vi "Teleop.vi"(10 "Match Info":T1={"Autonomous Elapsed Seconds"=0.0, "TeleOp Elapsed Seconds"=0.0, "Disabled Elapsed Seconds"=0.0, "Visited Autonomous"=FALSE, "Visited TeleOp"=FALSE, "Visited Disabled"=FALSE, "Autonomous Settings"={"Autonomous Style"=enum."Independent", "VI Refnum"=refnum}}, 11 "Call Context":T2) -> ()   [LabVIEW 2013]
doc: "This VI is called for each TeleOp packet received from the DS where the robot is not disabled. It is often used to read from the joysticks and update I/O or to update setpoints for timed control loops. It should complete and return within 20 milliseconds or it may miss DS packets."
uses:
  <vilib>/Rock Robotics/WPI/DriverStation/WPI_DriverStationDerivedRobotMode.ctl
  <vilib>/Rock Robotics/WPI/DriverStation/WPI_DriverStationMatch Info.ctl
  Robot Global Data.vi
  <vilib>/Rock Robotics/WPI/Solenoid/Deprecated/WPI_SolenoidSetBool.vi
  Angle.vi
  <vilib>/Rock Robotics/WPI/Joystick/WPI_JoystickGetSetRefNum.vi
  <vilib>/Rock Robotics/WPI/RobotDrive/WPI_RobotDriveGetSetRefNum.vi
panel:
  in  "Speed":dbl=0.5 format="%#_13g"
  out "Distance 2":dbl
  out "Rate 2":dbl
  out "Rate 1":dbl
  out "Distance 1":dbl
  out "Numeric 1":dbl(slide) scale=0.0..100.0
  out "Boolean 2":bool
  out "Boolean 1":bool
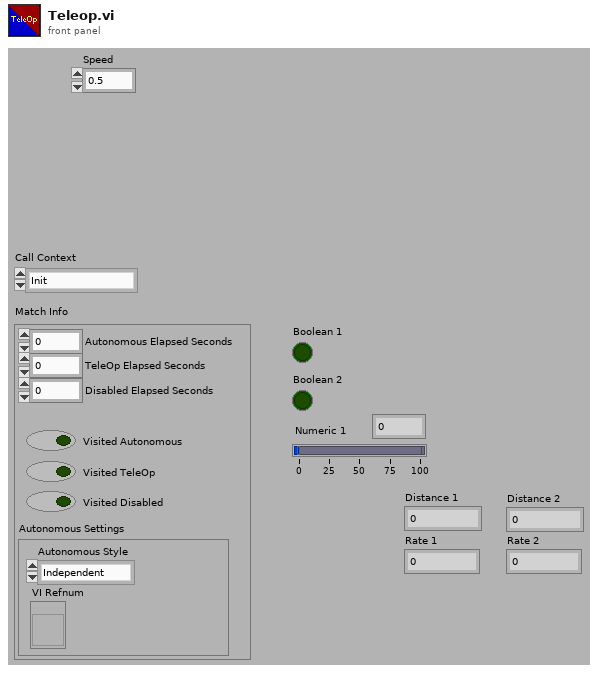
[diagram p1: front panel]
types:
  T1 = typedef "WPI_DriverStationMatch Info.ctl" = cluster{"Autonomous Elapsed Seconds":dbl, "TeleOp Elapsed Seconds":dbl, "Disabled Elapsed Seconds":dbl, "Visited Autonomous":bool, "Visited TeleOp":bool, "Visited Disabled":bool, "Autonomous Settings":cluster{"Autonomous Style":enum16{"Iterative", "Independent"}, "VI Refnum":refnum<vi>}}
  T2 = typedef "WPI_DriverStationDerivedRobotMode.ctl" = enum16{"Init", "Execute", "Stop"}
  T3 = typedef "WPI_RobotDriveDevRef.ctl" = cluster{"DevStatus":errorcluster, "Motors[]":T4[], "Square Inputs":bool, "Max Output":dbl, "Isochronous":bool}
  T4 = typedef "WPI_MotorControlDeviceRef.ctl" = cluster{"DeviceStatus":errorcluster, "Type":enum16{"PWM", "CAN"}, "PWM":cluster{"Digital Module":T5, "PWM Channel":T6, "DeadBand":T7}, "CAN":cluster{"Device Number":u8, "Control Mode":T8, "Semaphore":T9, "Max Vout":dbl}, "Invert":bool, "TransformRef":T10, "InvTransformRef":T10}
  T5 = typedef "FPGA_TypedefDigitalModule.ctl" = enum16{"Digital Module 1", "Digital Module 2"}
  T6 = typedef "FPGA_DIOPWMChannel.ctl" = enum8{"PWM 1", "PWM 2", "PWM 3", "PWM 4", "PWM 5", "PWM 6", "PWM 7", "PWM 8", "PWM 9", "PWM 10", "Invalid"}
  T7 = typedef "WPI_PWMDeadband.ctl" = cluster{"Name":string, "maxPositivePwm":i32, "minPositivePwm":i32, "centerPwm":i32, "maxNegativePwm":i32, "minNegativePwm":i32, "angularRange":u16}
  T8 = typedef "WPI_CANJaguar_ControlMode.ctl" = enum8{"Percent VBus", "Current", "Speed", "Position", "Voltage"}
  T9 = typedef "Semaphore RefNum" = refnum<k1>
  T10 = typedef "WPI_PWMTransform_ConPane.ctl" = refnum<vi>
  T11 = typedef "WPI_JoystickDevRef.ctl" = cluster{"Device":T12}
  T12 = typedef "WPI_JoystickDeviceEnum.ctl" = enum16{"USB 1", "USB 2", "USB 3", "USB 4", "Kinect 1", "Kinect 2"}
  T13 = typedef "WPI_JoystickButtonState.ctl" = cluster{"Button 1":bool, "Button 2":bool, "Button 3":bool, "Button 4":bool, "Button 5":bool, "Button 6":bool, "Button 7":bool, "Button 8":bool, "Button 9":bool, "Button 10":bool, "Button 11":bool, "Button 12":bool}
  T14 = cluster{"axis 1 (x)":dbl, "axis 2 (y)":dbl, "axis 3 (throttle)":dbl, "axis 4":dbl, "axis 5":dbl, "axis 6":dbl}
  T15 = typedef "WPI_SolenoidDevRef.ctl" = cluster{"DevStatus":errorcluster, "Solenoid Module":T16, "Forward Solenoid Channel":T17, "Reverse Solenoid Channel":T17}
  T16 = typedef "FPGA_TypedefSolenoidModule.ctl" = enum16{"Solenoid Module 1", "Solenoid Module 2"}
  T17 = typedef "WPI_SolenoidChannel.ctl" = enum8{"Solenoid 1", "Solenoid 2", "Solenoid 3", "Solenoid 4", "Solenoid 5", "Solenoid 6", "Solenoid 7", "Solenoid 8", "Invalid"}
  T18 = typedef "WPI_EncoderDevRef.ctl" = cluster{"DevStatus":errorcluster, "EncoderIndex":T19, "CounterIndex":T20, "DistancePerCount":dbl, "Decoding Type":T21}
  T19 = typedef "FPGA_EncoderIdx.ctl" = enum8{"Enc 0", "Enc 1", "Enc 2", "Enc 3", "Invalid"}
  T20 = typedef "FPGA_CounterCtrSystemIndex.ctl" = enum8{"Ctr 0", "Ctr 1", "Ctr 2", "Ctr 3", "Ctr 4", "Ctr 5", "Ctr 6", "Ctr 7", "Invalid"}
  T21 = typedef "WPI_EncoderType.ctl" = enum16{"1x", "2x", "4x"}
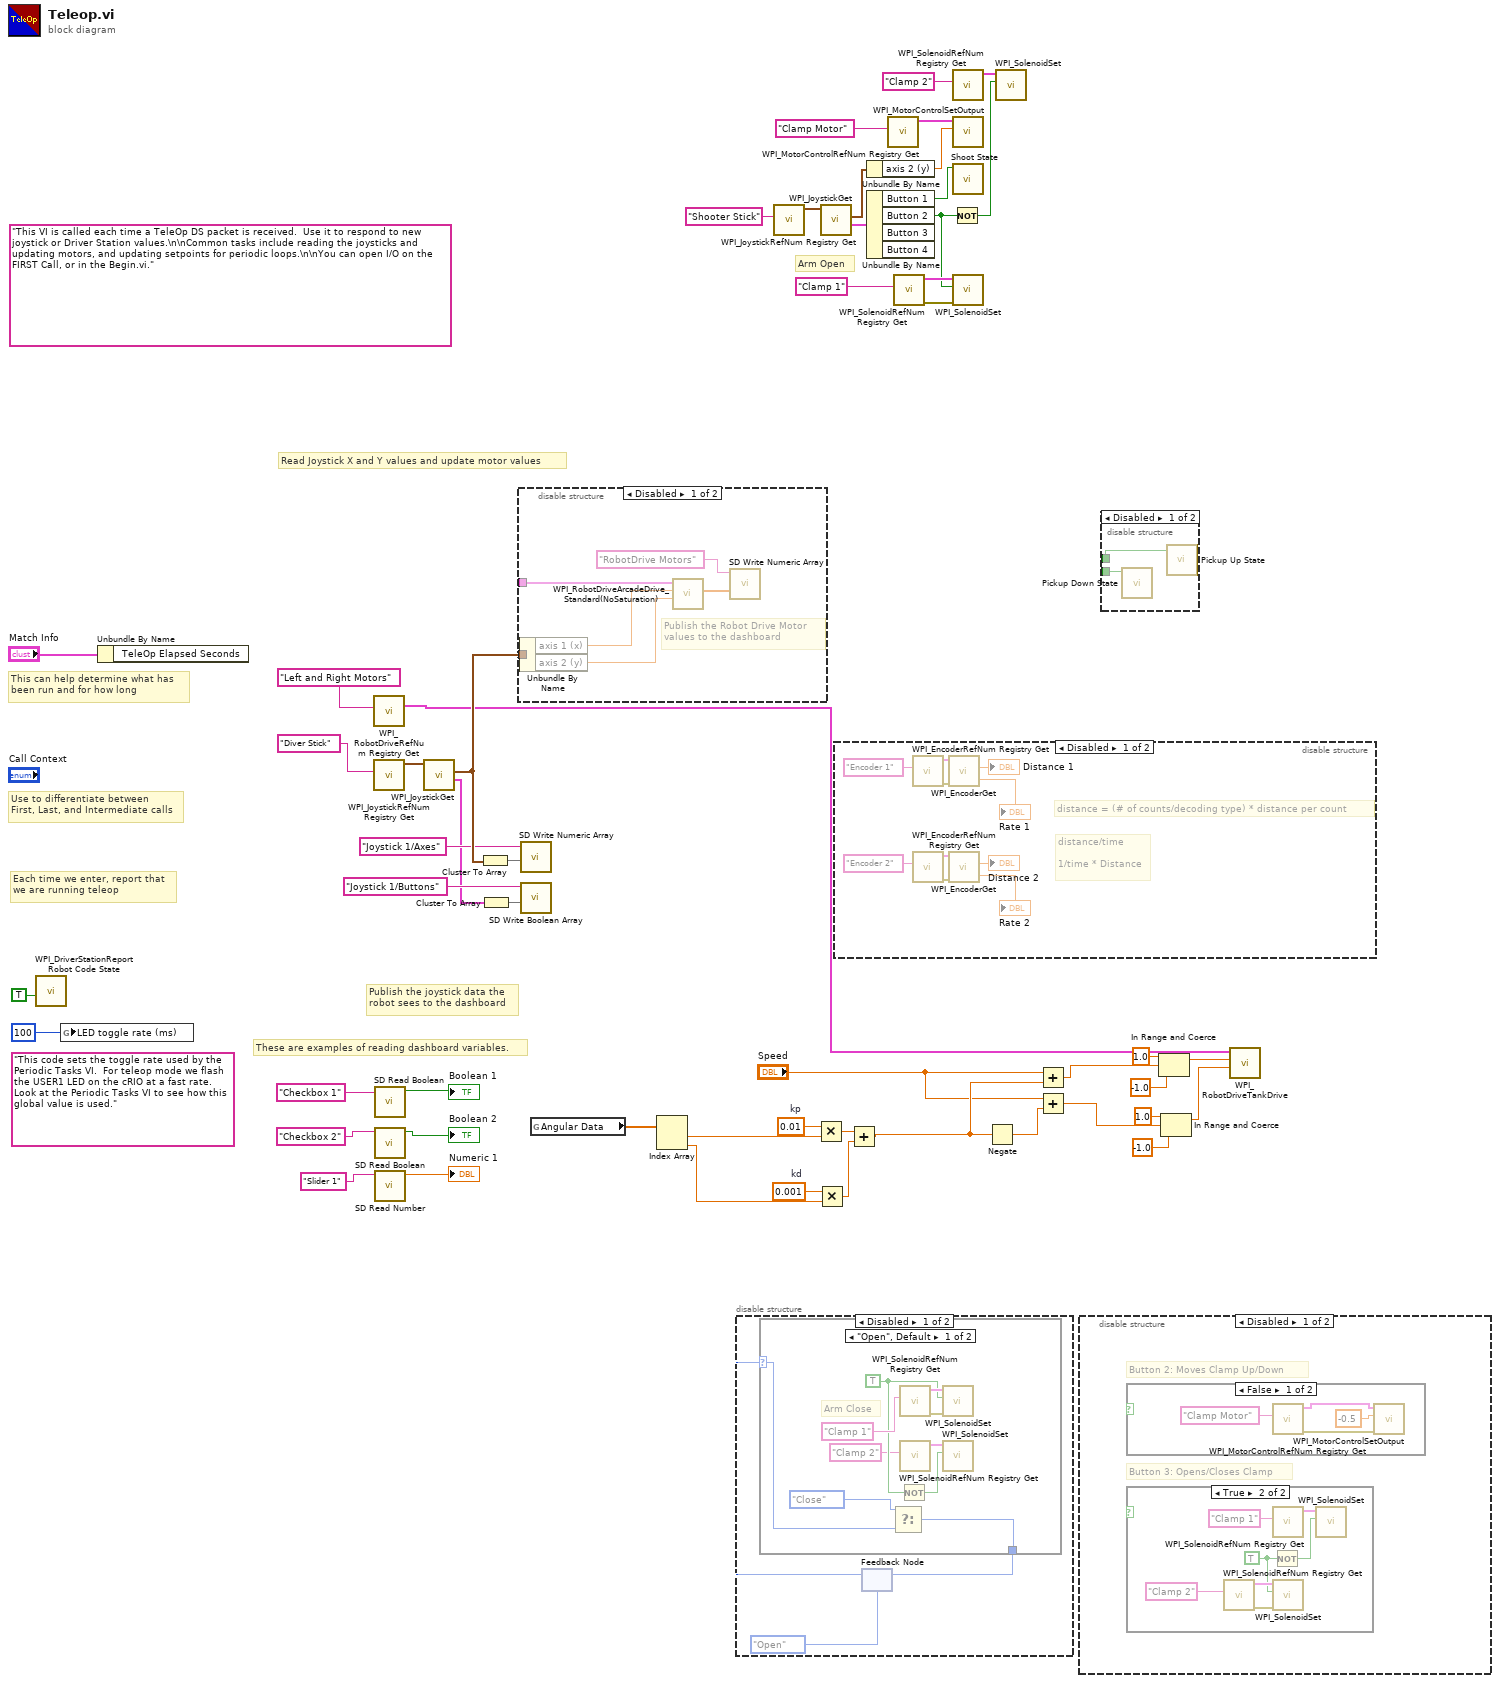
[diagram p0: block diagram]
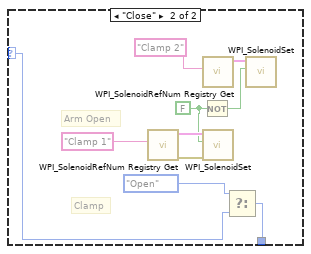
[diagram p5: hidden frame]
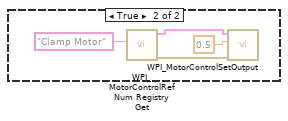
[diagram p8: hidden frame]
diagram:
  w15 = 0.001  # kd
  w19 = 0.01  # kp
  (unwired) "This code sets the toggle rate used by the Periodic Tasks VI.  For teleop mode we flash the USER1 LED on the cRIO at a fast rate.  Look at the Periodic Tasks VI to see how this global value is used."
  (unwired) "This VI is called each time a TeleOp DS packet is received.  Use it to respond to new joystick or Driver Station values.\n\nCommon tasks include reading the joysticks and updating motors, and updating setpoints for periodic loops.\n\nYou can open I/O on the FIRST Call, or in the Begin.vi."
  # "Arm Open"
  # "These are examples of reading dashboard variables."
  # "Publish the joystick data the\nrobot sees to the dashboard"
  # "Each time we enter, report that\nwe are running teleop"
  # "Use to differentiate between\nFirst, Last, and Intermediate calls"
  # "This can help determine what has\nbeen run and for how long"
  # "Read Joystick X and Y values and update motor values"
  n1 = call <vilib>:"WPI_DriverStationReport Robot Code State.vi"("TeleOp"=TRUE ("Autonomous")) -> ()  [unwired: 10 in, 1 out]
  n2 = global write "Robot Global Data.vi" "LED toggle rate (ms)"(u32 100 ("LED ms toggle rate")) -> ()
  n3 = Unbundle By Name("Match Info") -> ()  [unwired: 1 out]
  n4 = call <vilib>:"WPI_RobotDriveRefNum Registry Get.vi"("refnum name"="Left and Right Motors") -> ("RobotDriveDevRef"=w18:T3)  [unwired: 1 in, 9 out]
  n5 = call <vilib>:"WPI_JoystickRefNum Registry Get.vi"("refnum name"="Diver Stick") -> ("JoystickDevRef"=w49:T11)  [unwired: 1 in, 9 out]
  n6 = call <vilib>:"SD Read Boolean.vi"("Name"="Checkbox 1" ("refnum name")) -> ("Boolean"=→"Boolean 1":bool)  [unwired: 8 in, 2 out]
  n7 = call <vilib>:"SD Read Boolean.vi"("Name"="Checkbox 2" ("refnum name")) -> ("Boolean"=→"Boolean 2":bool)  [unwired: 8 in, 2 out]
  n8 = call <vilib>:"SD Read Number.vi"("Name"="Slider 1" ("refnum name")) -> ("Numeric"=→"Numeric 1":dbl)  [unwired: 8 in, 2 out]
  n9 = call <vilib>:"WPI_JoystickGet.vi"("JoystickDevRef"=w49) -> ("Buttons"=w33:T13, "Axes"=w44:T14)  [unwired: 1 in, 4 out]
  n10 = Cluster To Array(cluster=w44) -> (array=w43:dbl[])
  n11 = Cluster To Array(cluster=w33) -> (array=w46:bool[])
  n12 = disable-structure shown="Disabled" {
    disable-tunnel: w44 -> [w58 _]
    disable-tunnel: _ -> [w55 _]
    frame Disabled {
      # "Publish the Robot Drive Motor\nvalues to the dashboard"
      n13 = Unbundle By Name(w58) -> ("axis 1 (x)"=w56:dbl, "axis 2 (y)"=w57:dbl)
      n14 = call <vilib>:"WPI_RobotDriveArcadeDrive_Standard(NoSaturation).vi"("Y axis value"=w57, "X axis value"=w56, "RobotDriveDevRef"=w55) -> ("Motor Values"=w53:dbl[])  [unwired: 1 in, 7 out]
      n15 = call <vilib>:"SD Write Numeric Array.vi"("Numeric Array"=w53, "Name"="RobotDrive Motors") -> ()  [unwired: 8 in, 2 out]
    }
    frame Enabled {
    }
  }
  n16 = call <vilib>:"SD Write Numeric Array.vi"("Numeric Array"=w43, "Name"="Joystick 1/Axes") -> ()  [unwired: 8 in, 2 out]
  n17 = call <vilib>:"SD Write Boolean Array.vi"("Boolean Array"=w46, "Name"="Joystick 1/Buttons") -> ()  [unwired: 8 in, 2 out]
  n18 = global read "Angle.vi" "Angular Data"() -> (w16:dbl[])
  n19 = Index Array(array=w16) -> (element #1=w11:dbl, element #2=w10:dbl)  [unwired: 2 in]
  n20 = disable-structure shown="Disabled" {
    frame Disabled {
      n21 = feedback #1(enum16{"Open", "Close"}."Open") -> (w60:enum16{"Open", "Close"})
      n22 = case shown="\"Open\", Default" w60 {
        selector: w60 -> [w63 w73]
        tunnel: [w62 w72] -> w59
        frame "Open", Default {
          w68 = TRUE
          # "Arm Close"
          n23 = Select(t=enum16{"Open", "Close"}."Close", f=w63) -> (s? t:f=w62:enum16{"Open", "Close"})  [unwired: 1 in]
          n24 = Not(x=w68) -> (.not. x?=w66:bool)
          n25 = call <vilib>:"WPI_SolenoidRefNum Registry Get.vi"("refnum name"="Clamp 1") -> ("error out"=w69:errorcluster, "SolenoidDevRef"=w70:T15)  [unwired: 9 in]
          n26 = call <vilib>:"WPI_SolenoidRefNum Registry Get.vi"("refnum name"="Clamp 2") -> ("SolenoidDevRef"=w67:T15)  [unwired: 9 in, 1 out]
          n27 = call-poly <vilib>:"WPI_SolenoidSet.vi"("error in (no error)"=w69, "Value"=w68, "SolenoidDevRef"=w70) -> ()  [unwired: 7 in, 2 out]
          n28 = call-poly <vilib>:"WPI_SolenoidSet.vi"("Value"=w66, "SolenoidDevRef"=w67) -> ()  [unwired: 8 in, 2 out]
        }
        frame "Close" {
          w75 = FALSE ("x")
          # "Arm Open"
          # "Clamp"
          n29 = call <vilib>:"WPI_SolenoidRefNum Registry Get.vi"("refnum name"="Clamp 1") -> ("error out"=w79:errorcluster, "SolenoidDevRef"=w80:T15)  [unwired: 9 in]
          n30 = Not(x=w75) -> (.not. x?=w76:bool)
          n31 = call <vilib>:"WPI_SolenoidRefNum Registry Get.vi"("refnum name"="Clamp 2") -> ("SolenoidDevRef"=w78:T15)  [unwired: 9 in, 1 out]
          n32 = call-poly <vilib>:"WPI_SolenoidSet.vi"("error in (no error)"=w79, "Value"=w75, "SolenoidDevRef"=w80) -> ()  [unwired: 7 in, 2 out]
          n33 = Select(t=enum16{"Open", "Close"}."Open", f=w73) -> (s? t:f=w72:enum16{"Open", "Close"})  [unwired: 1 in]
          n34 = call-poly <vilib>:"WPI_SolenoidSet.vi"("Value"=w76, "SolenoidDevRef"=w78) -> ()  [unwired: 8 in, 2 out]
        }
      }
      n35 = feedback-in #1(w59) -> ()
    }
    frame Enabled {
    }
  }
  n36 = call <vilib>:"WPI_JoystickRefNum Registry Get.vi"("refnum name"="Shooter Stick") -> ("JoystickDevRef"=w35:T11)  [unwired: 1 in, 9 out]
  n37 = Multiply(x=w19, y=w11) -> (x*y=w17:dbl)
  n38 = Multiply(x=w15, y=w10) -> (x*y=w14:dbl)
  n39 = call <vilib>:"WPI_JoystickGet.vi"("JoystickDevRef"=w35) -> ("Buttons"=w32:T13, "Axes"=w31:T14)  [unwired: 1 in, 4 out]
  n40 = disable-structure shown="Disabled" {
    frame Disabled {
      # "distance/time\n\n1/time * Distance"
      # "distance = (# of counts/decoding type) * distance per count"
      n41 = call <vilib>:"WPI_EncoderRefNum Registry Get.vi"("refnum name"="Encoder 1") -> ("error out"=w90:errorcluster, "EncoderDevRef"=w89:T18)  [unwired: 9 in]
      n42 = call <vilib>:"WPI_EncoderRefNum Registry Get.vi"("refnum name"="Encoder 2") -> ("error out"=w84:errorcluster, "EncoderDevRef"=w82:T18)  [unwired: 9 in]
      n43 = call <vilib>:"WPI_EncoderGet.vi"("error in (no error)"=w90, "EncoderDevRef"=w89) -> ("Distance"=→"Distance 1":dbl, "Rate"=→"Rate 1":dbl)  [unwired: 4 in, 4 out]
      n44 = call <vilib>:"WPI_EncoderGet.vi"("error in (no error)"=w84, "EncoderDevRef"=w82) -> ("Distance"=→"Distance 2":dbl, "Rate"=→"Rate 2":dbl)  [unwired: 4 in, 4 out]
    }
    frame Enabled {
    }
  }
  n45 = Add(x=w17, y=w14) -> (x+y=w8:dbl)
  n46 = Unbundle By Name(w31) -> ("axis 2 (y)"=w27:dbl)
  n47 = Unbundle By Name(w32) -> ("Button 1"=w30:bool, "Button 2"=w20:bool)  [unwired: 2 out]
  n48 = call <vilib>:"WPI_MotorControlRefNum Registry Get.vi"("refnum name"="Clamp Motor") -> ("MotorControlDevRef"=w28:T4)  [unwired: 9 in, 1 out]
  n49 = call <vilib>:"WPI_SolenoidRefNum Registry Get.vi"("refnum name"="Clamp 1") -> ("error out"=w24:errorcluster, "SolenoidDevRef"=w25:T15)  [unwired: 9 in]
  n50 = Not(x=w20) -> (.not. x?=w21:bool)
  n51 = call <vilib>:"WPI_SolenoidRefNum Registry Get.vi"("refnum name"="Clamp 2") -> ("SolenoidDevRef"=w23:T15)  [unwired: 9 in, 1 out]
  n52 = call <vilib>:"WPI_MotorControlSetOutput.vi"("Output"=w27, "MotorControlDevRef"=w28) -> ()  [unwired: 7 in, 3 out]
  n53 = call "Shoot State.vi"("Trigger"=w30) -> ()  [unwired: 9 in, 2 out]
  n54 = call-poly <vilib>:"WPI_SolenoidSet.vi"("error in (no error)"=w24, "Value"=w20, "SolenoidDevRef"=w25) -> ()  [unwired: 7 in, 2 out]
  n55 = Negate(x=w8) -> (-x=w9:dbl)
  n56 = call-poly <vilib>:"WPI_SolenoidSet.vi"("Value"=w21, "SolenoidDevRef"=w23) -> ()  [unwired: 8 in, 2 out]
  n57 = Add(x="Speed", y=w8) -> (x+y=w2:dbl)
  n58 = Add(x="Speed", y=w9) -> (x+y=w7:dbl)
  n59 = disable-structure shown="Disabled" {
    frame Disabled {
      # "Button 3: Opens/Closes Clamp"
      # "Button 2: Moves Clamp Up/Down"
      n60 = case shown="False" {
        selector: _ -> [_ _]
        frame False {
          n61 = call <vilib>:"WPI_MotorControlRefNum Registry Get.vi"("refnum name"="Clamp Motor") -> ("error out"=w101:errorcluster, "MotorControlDevRef"=w100:T4)  [unwired: 9 in]
          n62 = call <vilib>:"WPI_MotorControlSetOutput.vi"("error in (no error)"=w101, "Output"=-0.5, "MotorControlDevRef"=w100) -> ()  [unwired: 6 in, 3 out]
        }
        frame True {
          n63 = call <vilib>:"WPI_MotorControlRefNum Registry Get.vi"("refnum name"="Clamp Motor") -> ("error out"=w105:errorcluster, "MotorControlDevRef"=w104:T4)  [unwired: 9 in]
          n64 = call <vilib>:"WPI_MotorControlSetOutput.vi"("error in (no error)"=w105, "Output"=0.5, "MotorControlDevRef"=w104) -> ()  [unwired: 6 in, 3 out]
        }
      }
      n65 = case shown="True" {
        selector: _ -> [_ _]
        frame False {
        }
        frame True {
          w93 = TRUE
          n66 = call <vilib>:"WPI_SolenoidRefNum Registry Get.vi"("refnum name"="Clamp 2") -> ("error out"=w94:errorcluster, "SolenoidDevRef"=w95:T15)  [unwired: 9 in]
          n67 = Not(x=w93) -> (.not. x?=w92:bool)
          n68 = call <vilib>:"WPI_SolenoidRefNum Registry Get.vi"("refnum name"="Clamp 1") -> ("SolenoidDevRef"=w97:T15)  [unwired: 9 in, 1 out]
          n69 = call-poly <vilib>:"WPI_SolenoidSet.vi"("error in (no error)"=w94, "Value"=w93, "SolenoidDevRef"=w95) -> ()  [unwired: 7 in, 2 out]
          n70 = call-poly <vilib>:"WPI_SolenoidSet.vi"("Value"=w92, "SolenoidDevRef"=w97) -> ()  [unwired: 8 in, 2 out]
        }
      }
    }
    frame Enabled {
    }
  }
  n71 = disable-structure shown="Disabled" {
    disable-tunnel: _ -> [w108 _]
    disable-tunnel: _ -> [w107 _]
    frame Disabled {
      n72 = call "Pickup Down State.vi"("Trigger"=w107) -> ()  [unwired: 11 in]
      n73 = call "Pickup Up State.vi"("Trigger"=w108) -> ()  [unwired: 11 in]
    }
    frame Enabled {
    }
  }
  n74 = In Range and Coerce(upper limit=1.0, x=w2, lower limit=-1.0) -> (coerced(x)=w4:dbl)  [unwired: 1 out]
  n75 = In Range and Coerce(upper limit=1.0, x=w7, lower limit=-1.0) -> (coerced(x)=w3:dbl)  [unwired: 1 out]
  n76 = call <vilib>:"WPI_RobotDriveTankDrive.vi"("Right axis value"=w3, "Left axis value"=w4, "RobotDriveDevRef"=w18) -> ()  [unwired: 6 in, 3 out]
